vi "ui_loop_message_handling.vi"(8 "error in (no error)":errorcluster caption="错误输入（无错误）", 9 "UI Control Refs Cluster":T1 caption="UI控件引用簇", 10 "User Event - Stop":refnum<user-event>, 11 "UI Message Queue Ref":refnum<queue> caption="UI消息队列引用") -> (0 "error out":errorcluster caption="错误输出")   [LabVIEW 2015]
uses:
  support_vis/message_queue/message_cluster.ctl
  type_definitions/ui_data.ctl
  type_definitions/shared_variables.ctl
  globals/global_all_ui_loop_stop.vi
  globals/global_configuration_options.vi
  globals/global_ui_stream_and_variable_connections.vi
  support_vis/message_queue/message_queue.lvlib
  support_vis/user_event_stop/user_event_stop.lvlib
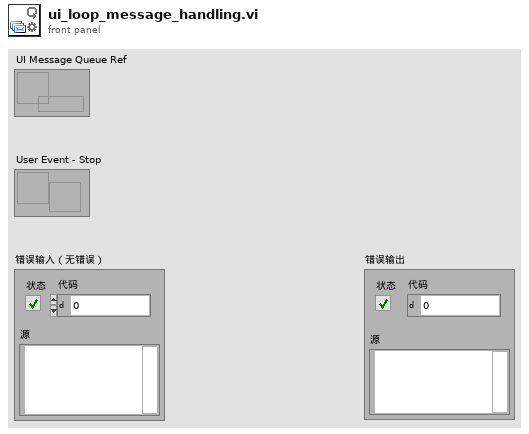
[diagram p1: front panel]
types:
  T1 = typedef "ui_data.ctl" = cluster{"Connected? Ref":refnum<vi>, "Controller Address Ref":refnum<vi>, "Error Infomation Ref":refnum<vi>, "Scan Engine Period (ms) Ref":refnum<vi>, "Number of Data Files Ref":refnum<vi>, "System Time Ref":refnum<vi>, "Free Memory Ref":refnum<vi>, "Device Tree Ref":refnum<vi>, "Controller Working Status Ref":refnum<vi>, "Connect to RT":refnum<vi>, "Exit":refnum<vi>, "Tab Ref":refnum<vi>, "Live Data Ref":refnum<vi>, "Resource Utilization (%) Ref":refnum<vi>}
  T2 = enum8{"Enabled", "Disabled", "Disabled and Grayed Out"}
  T3 = typedef "message_queue.lvlib/message_cluster.ctl" = cluster{"Message":string, "Message Data":variant}
  T4 = cluster{"Left Cell String":string, "Child Text":string[], "Child Tag":string, "Item Indent":i32, "Child Only?":bool, "Glyph Index":i32}[]
  T5 = typedef "shared_variables.ctl" = cluster{"System Time":timestamp, "CPU 1 Usage":dbl, "CPU 2 Usage":dbl, "Driver Space":dbl, "Free Memory":dbl, "Scan Engine Period (ms)":u32, "Number of Data Files":u32}
  T6 = cluster{"CPU 1 Usage":dbl, "CPU 2 Usage":dbl, "Driver Space":dbl}
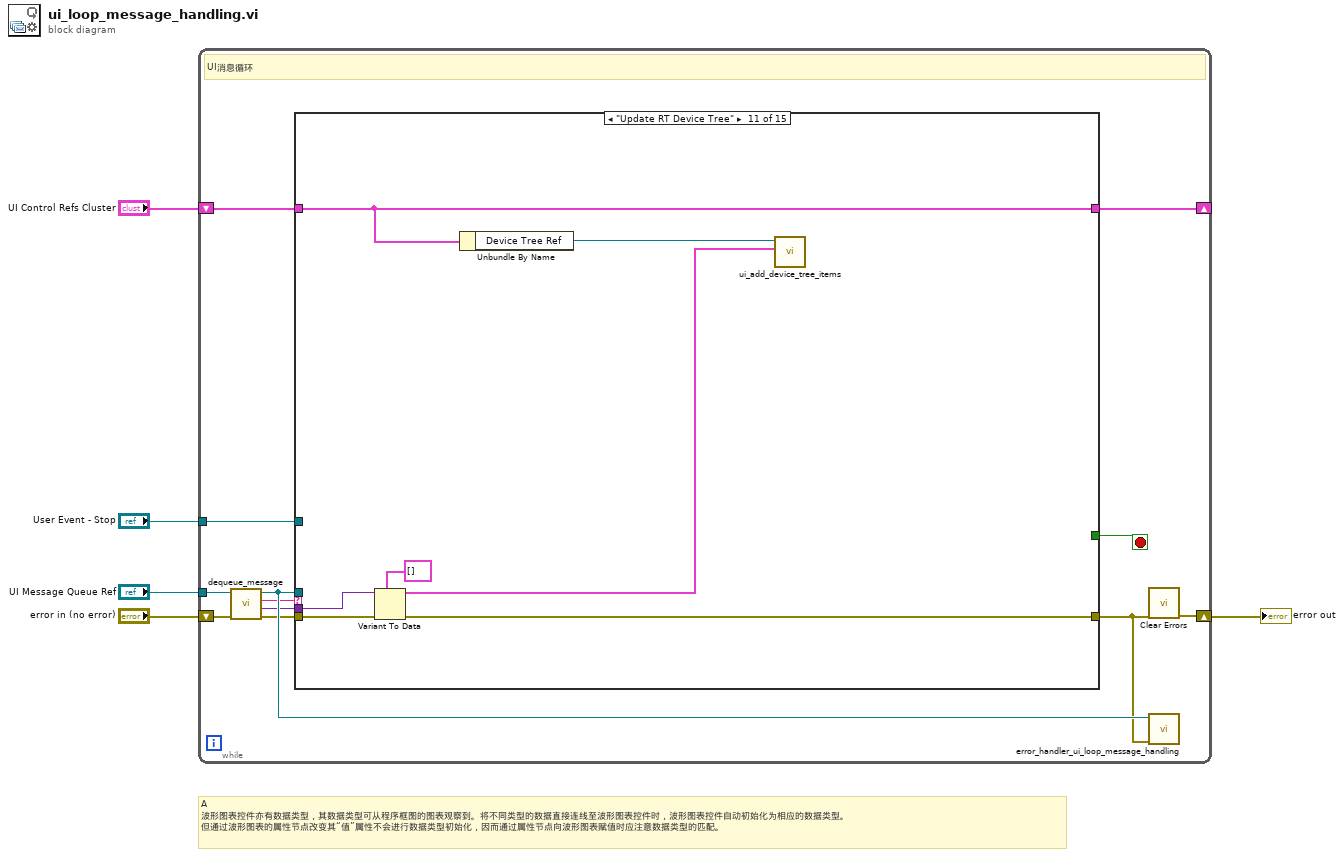
[diagram p0: block diagram]
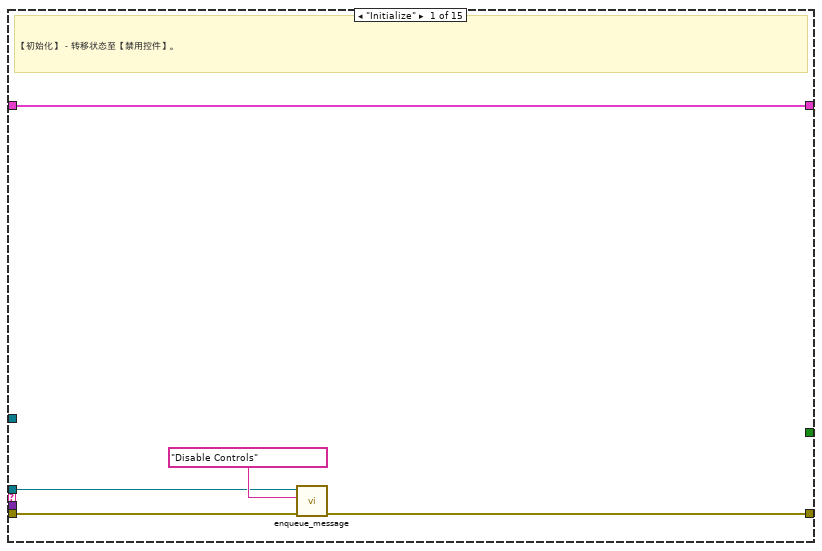
[diagram p2: hidden frame]
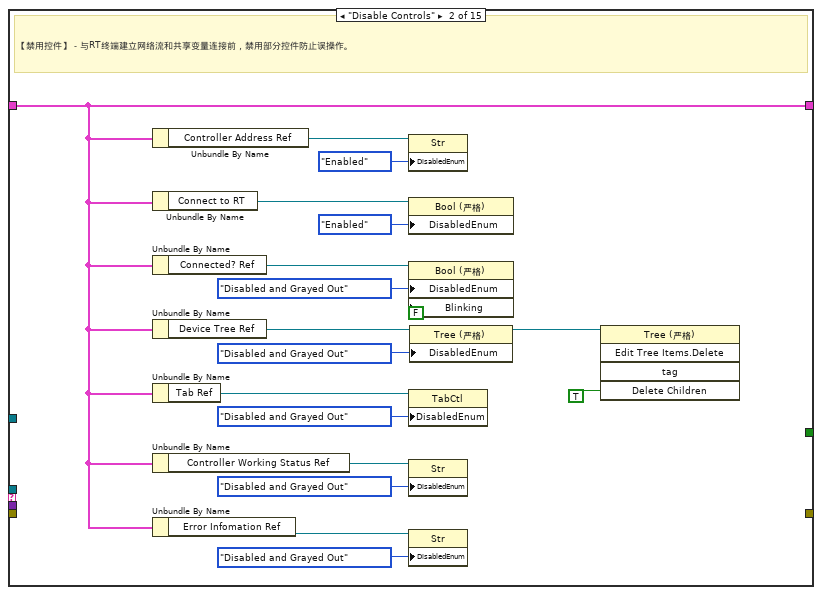
[diagram p3: hidden frame]
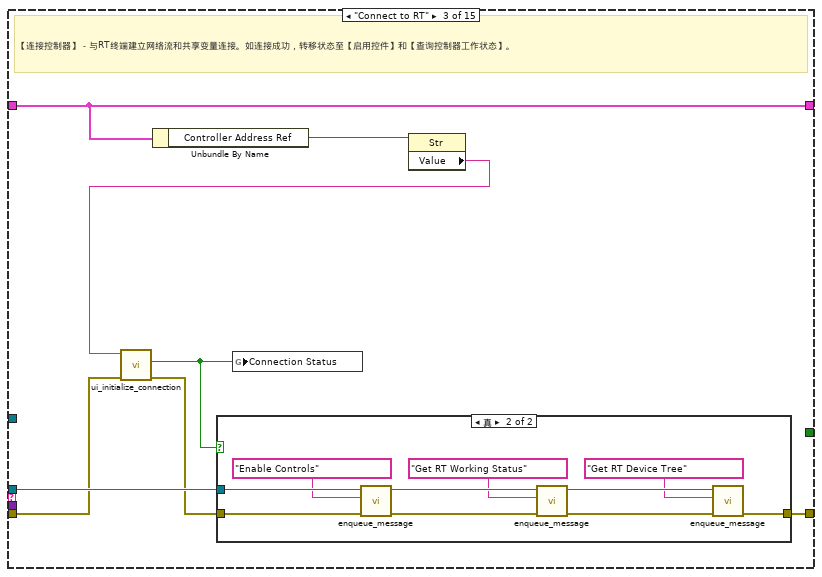
[diagram p4: hidden frame]
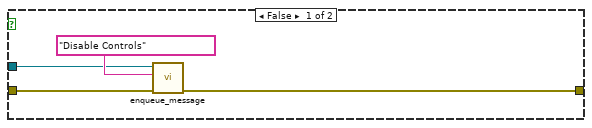
[diagram p5: hidden frame]
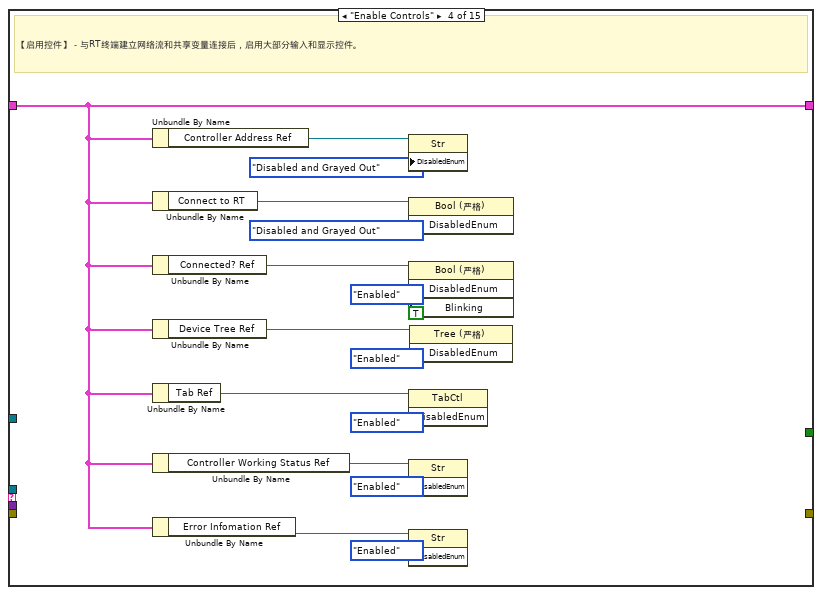
[diagram p6: hidden frame]
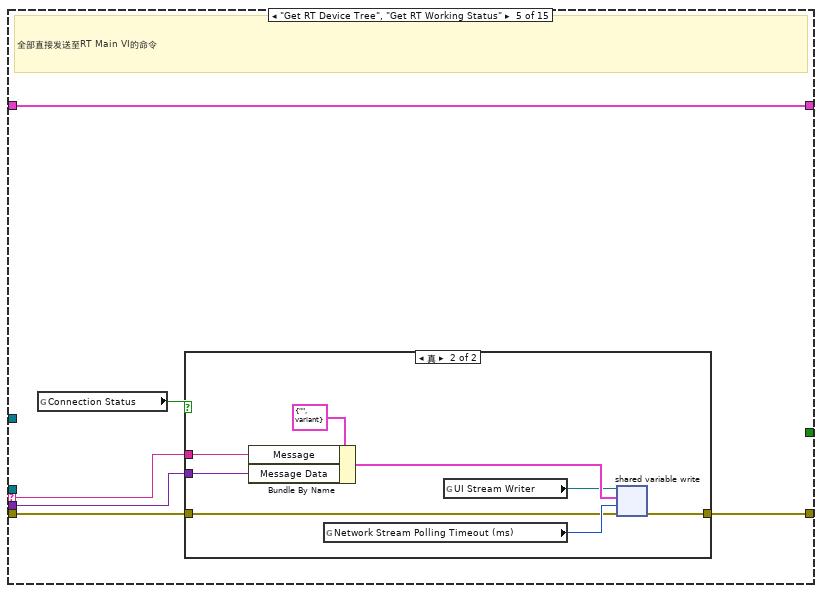
[diagram p7: hidden frame]
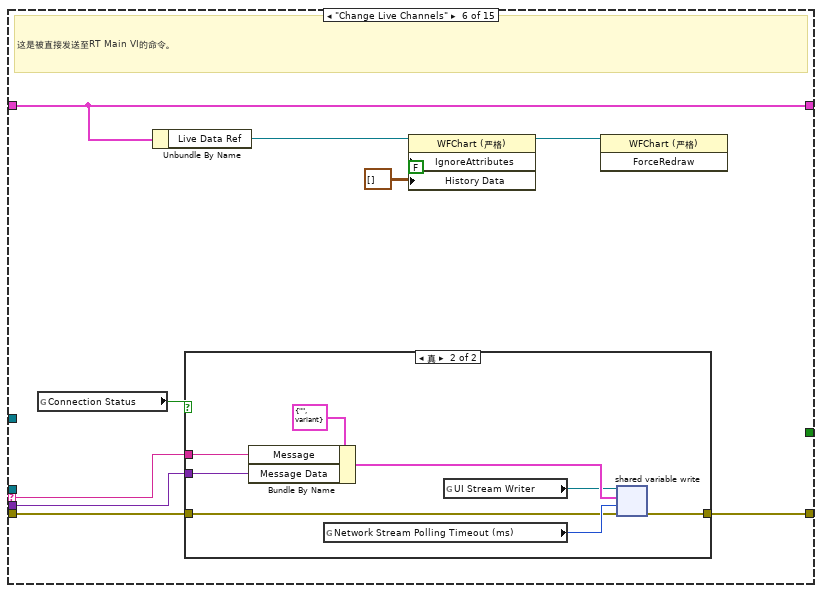
[diagram p9: hidden frame]
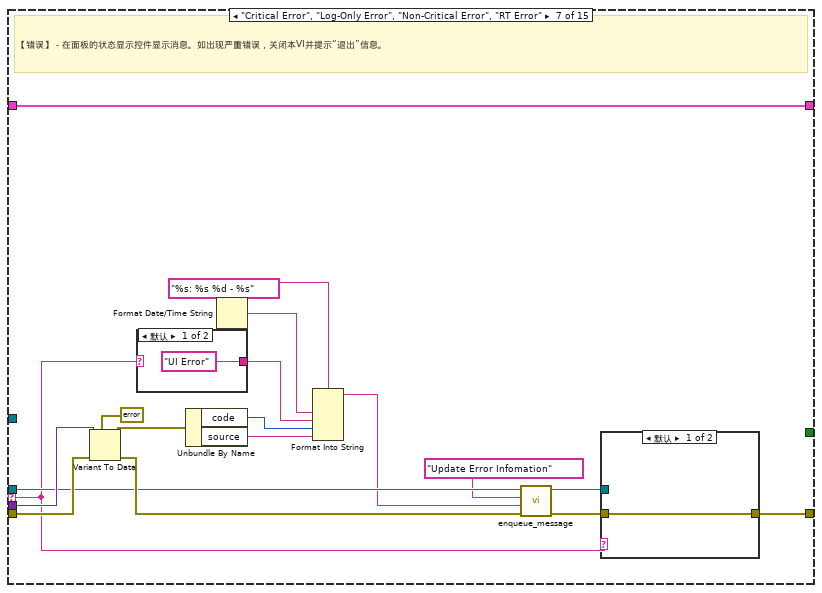
[diagram p11: hidden frame]
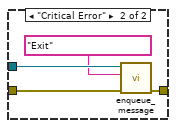
[diagram p13: hidden frame]
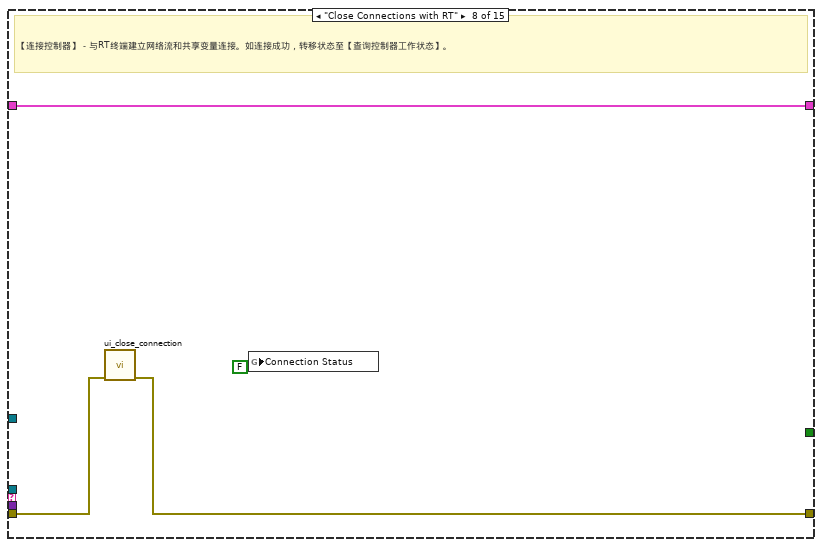
[diagram p14: hidden frame]
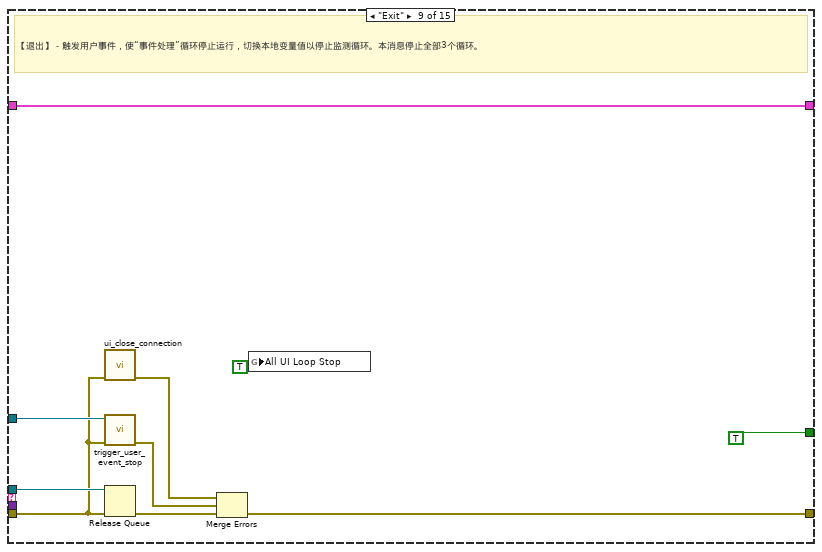
[diagram p15: hidden frame]
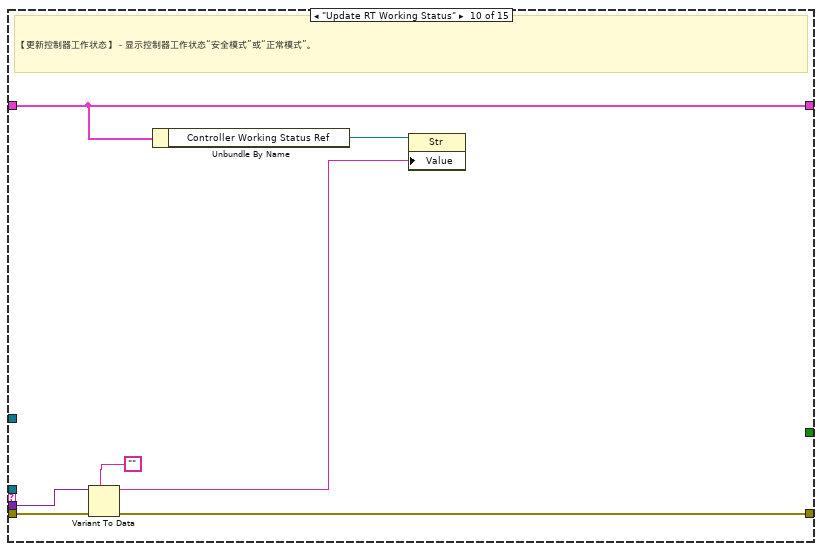
[diagram p16: hidden frame]
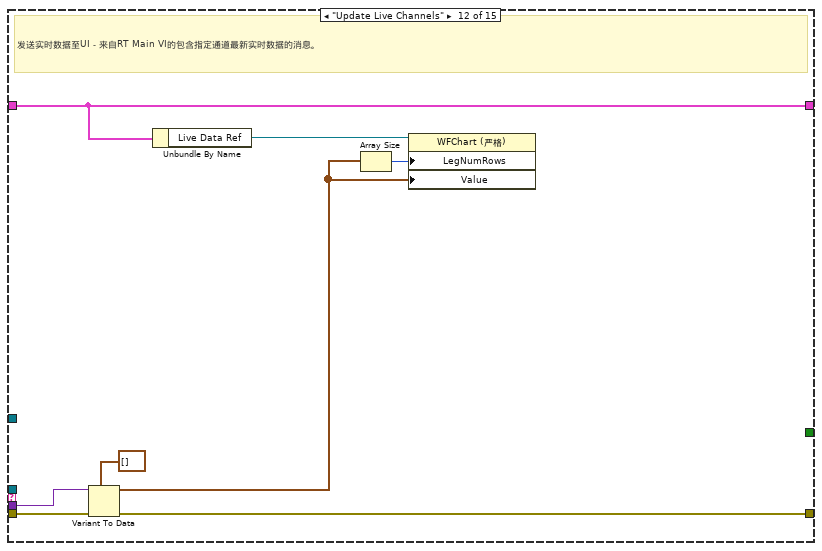
[diagram p17: hidden frame]
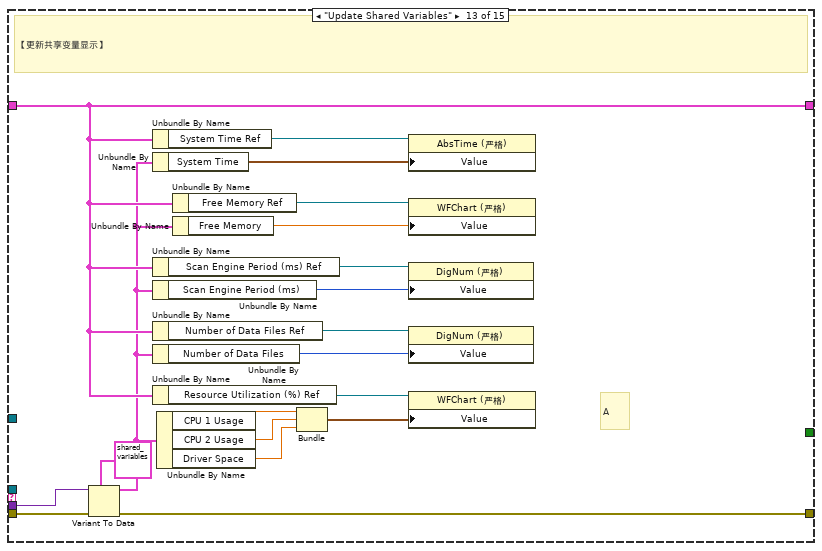
[diagram p18: hidden frame]
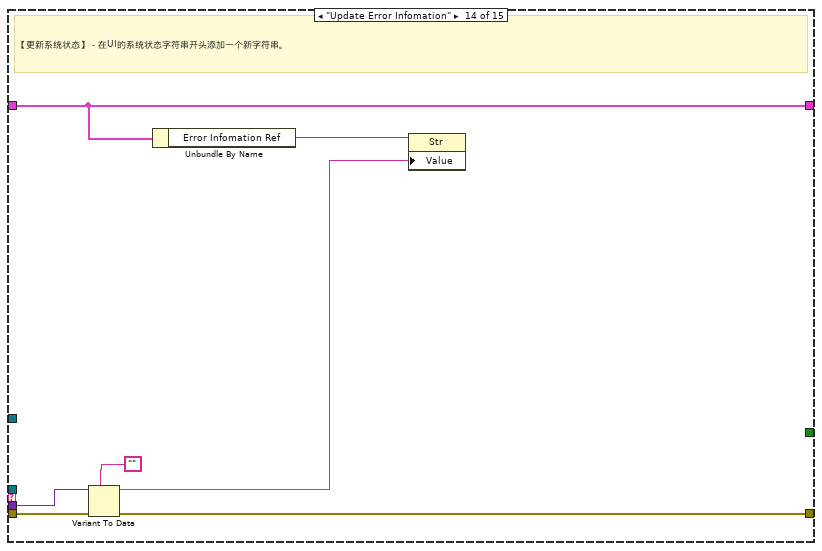
[diagram p19: hidden frame]
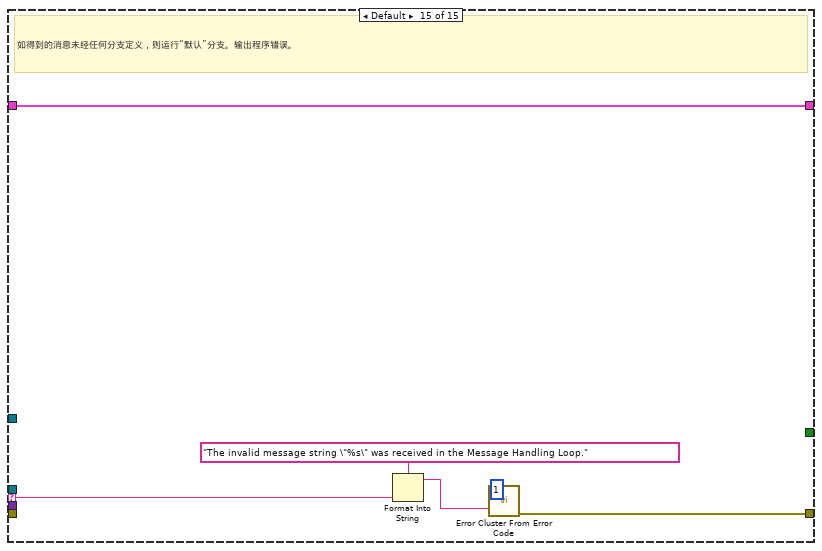
[diagram p20: hidden frame]
diagram:
  # "A\n波形图表控件亦有数据类型，其数据类型可从程序框图的图表观察到。将不同类型的数据直接连线至波形图表控件时，波形图表控件自动初始化为相应的数据类型。\n但通过波形图表的属性节点改变其“值”属性不会进行数据类型初始化，因而通过属性节点向波形图表赋值时应注意数据类型的匹配。"
  n1 = while {
    tunnel: "UI Message Queue Ref" -> [w10]
    tunnel: "User Event - Stop" -> [w15]
    shift-right: [w6] -> w1
    shift-left: "error in (no error)" -> [w14]
    shift-right: [w8] -> _
    shift-left: "UI Control Refs Cluster" -> [w9]
    stop <- w16 stop-if-true
    # "UI消息循环"
    n2 = call "dequeue_message.vi"("error in (no error)"=w14, "Message Queue"=w10) -> ("error out"=w13:errorcluster, "Message Data"=w11:variant, "Message"=w12:string, "dup Message Queue"=w17:refnum<queue>)  [unwired: 6 in]
    n3 = case "Message Cases" shown="\"Update RT Device Tree\"" w12 {
      selector: w12 -> [_ _ _ _ w81 w100 w114 _ _ _ _ _ _ _ w204]
      tunnel: w17 -> [w18 _ w45 _ _ _ w118 _ w146 _ _ _ _ _ _]
      tunnel: w13 -> [w21 _ w43 _ w84 w103 w128 w140 w144 w158 w164 w173 w192 w199 _]
      tunnel: [w19 _ w48 _ w83 w102 w129 w139 w150 w157 w163 w172 w191 w198 w202] -> w7
      tunnel: [_ _ _ _ _ _ _ _ TRUE _ _ _ _ _ _] -> w16
      tunnel: w11 -> [_ _ _ _ w82 w101 w126 _ _ w156 w162 w171 w190 w197 _]
      tunnel: w15 -> [_ _ _ _ _ _ _ _ w149 _ _ _ _ _ _]
      tunnel: w9 -> [w22 w25 w47 w63 w79 w98 w130 w141 w148 w154 w165 w169 w177 w195 w200]
      tunnel: [w22 w25 w47 w63 w79 w98 w130 w141 w148 w154 w165 w169 w177 w195 w200] -> w8
      frame "Initialize" {
        # "【初始化】－转移状态至【禁用控件】。"
        n4 = call "enqueue_message.vi"("error in (no error)"=w21, "Message"="Disable Controls", "Message Queue"=w18) -> ("error out"=w19:errorcluster)  [unwired: 7 in, 1 out]
      }
      frame "Disable Controls" {
        # "【禁用控件】－与RT终端建立网络流和共享变量连接前，禁用部分控件防止误操作。"
        n5 = Unbundle By Name(w25) -> ("Controller Address Ref"=w40:refnum<vi>)
        n6 = Unbundle By Name(w25) -> ("Connect to RT"=w37:refnum<vi>)
        n7 = Unbundle By Name(w25) -> ("Connected? Ref"=w36:refnum<vi>)
        n8 = Unbundle By Name(w25) -> ("Device Tree Ref"=w33:refnum<vi>)
        n9 = Unbundle By Name(w25) -> ("Tab Ref"=w30:refnum<vi>)
        n10 = Unbundle By Name(w25) -> ("Controller Working Status Ref"=w29:refnum<vi>)
        n11 = Unbundle By Name(w25) -> ("Error Infomation Ref"=w26:refnum<vi>)
        n12 = property class="Str"(reference=w40, "DisabledEnum"=T2."Enabled" ("禁用")) -> ()  [unwired: 1 in, 2 out]
        n13 = property class="Bool (严格)"(reference=w37, "DisabledEnum"=T2."Enabled" ("禁用")) -> ()  [unwired: 1 in, 2 out]
        n14 = property class="Bool (严格)"(reference=w36, "DisabledEnum"=T2."Disabled and Grayed Out" ("禁用"), "Blinking"=FALSE ("闪烁")) -> ()  [unwired: 1 in, 2 out]
        n15 = property class="TabCtl"(reference=w30, "DisabledEnum"=T2."Disabled and Grayed Out" ("禁用")) -> ()  [unwired: 1 in, 2 out]
        n16 = property class="Str"(reference=w29, "DisabledEnum"=T2."Disabled and Grayed Out" ("禁用")) -> ()  [unwired: 1 in, 2 out]
        n17 = property class="Str"(reference=w26, "DisabledEnum"=T2."Disabled and Grayed Out" ("禁用")) -> ()  [unwired: 1 in, 2 out]
        n18 = property class="Tree (严格)"(reference=w33, "DisabledEnum"=T2."Disabled and Grayed Out" ("禁用")) -> (reference out=w24:refnum<vi>)  [unwired: 1 in, 1 out]
        n19 = invoke class="Tree (严格)" method="Edit Tree Items.Delete"(reference=w24, "Delete Children"=TRUE ("删除子项？")) -> ()  [unwired: 3 in, 5 out]
      }
      frame "Connect to RT" {
        # "【连接控制器】－与RT终端建立网络流和共享变量连接。如连接成功，转移状态至【启用控件】和【查询控制器工作状态】。"
        n20 = Unbundle By Name(w47) -> ("Controller Address Ref"=w46:refnum<vi>)
        n21 = property class="Str"(reference=w46) -> ("Value"=w44:string)  [unwired: 1 in, 2 out]
        n22 = call "ui_initialize_connection.vi"("error in (no error)"=w43, "Controller Address"=w44) -> ("error out"=w42:errorcluster, "Connected?"=w41:bool)  [unwired: 8 in]
        n23 = case shown="真" w41 {
          tunnel: [w52 w56] -> w48
          tunnel: w45 -> [w50 w62]
          tunnel: w42 -> [w49 w61]
          frame False {
            n24 = call "enqueue_message.vi"("error in (no error)"=w49, "Message"="Disable Controls", "Message Queue"=w50) -> ("error out"=w52:errorcluster)  [unwired: 7 in, 1 out]
          }
          frame True {
            n25 = call "enqueue_message.vi"("error in (no error)"=w61, "Message"="Enable Controls", "Message Queue"=w62) -> ("error out"=w59:errorcluster, "dup Message Queue"=w60:refnum<queue>)  [unwired: 7 in]
            n26 = call "enqueue_message.vi"("error in (no error)"=w59, "Message"="Get RT Working Status", "Message Queue"=w60) -> ("error out"=w58:errorcluster, "dup Message Queue"=w57:refnum<queue>)  [unwired: 7 in]
            n27 = call "enqueue_message.vi"("error in (no error)"=w58, "Message"="Get RT Device Tree", "Message Queue"=w57) -> ("error out"=w56:errorcluster)  [unwired: 7 in, 1 out]
          }
        }
        n28 = global write "global_all_ui_loop_stop.vi" "Connection Status"(w41) -> ()
      }
      frame "Enable Controls" {
        # "【启用控件】－与RT终端建立网络流和共享变量连接后，启用大部分输入和显示控件。"
        n29 = Unbundle By Name(w63) -> ("Controller Address Ref"=w78:refnum<vi>)
        n30 = Unbundle By Name(w63) -> ("Connect to RT"=w75:refnum<vi>)
        n31 = Unbundle By Name(w63) -> ("Connected? Ref"=w74:refnum<vi>)
        n32 = Unbundle By Name(w63) -> ("Device Tree Ref"=w71:refnum<vi>)
        n33 = Unbundle By Name(w63) -> ("Tab Ref"=w68:refnum<vi>)
        n34 = Unbundle By Name(w63) -> ("Controller Working Status Ref"=w67:refnum<vi>)
        n35 = Unbundle By Name(w63) -> ("Error Infomation Ref"=w64:refnum<vi>)
        n36 = property class="Str"(reference=w78, "DisabledEnum"=T2."Disabled and Grayed Out" ("禁用")) -> ()  [unwired: 1 in, 2 out]
        n37 = property class="Bool (严格)"(reference=w75, "DisabledEnum"=T2."Disabled and Grayed Out" ("禁用")) -> ()  [unwired: 1 in, 2 out]
        n38 = property class="Bool (严格)"(reference=w74, "DisabledEnum"=T2."Enabled" ("禁用"), "Blinking"=TRUE ("闪烁")) -> ()  [unwired: 1 in, 2 out]
        n39 = property class="TabCtl"(reference=w68, "DisabledEnum"=T2."Enabled" ("禁用")) -> ()  [unwired: 1 in, 2 out]
        n40 = property class="Str"(reference=w67, "DisabledEnum"=T2."Enabled" ("禁用")) -> ()  [unwired: 1 in, 2 out]
        n41 = property class="Str"(reference=w64, "DisabledEnum"=T2."Enabled" ("禁用")) -> ()  [unwired: 1 in, 2 out]
        n42 = property class="Tree (严格)"(reference=w71, "DisabledEnum"=T2."Enabled" ("禁用")) -> ()  [unwired: 1 in, 2 out]
      }
      frame "Get RT Device Tree", "Get RT Working Status" {
        # "全部直接发送至RT Main VI的命令"
        n43 = global read "global_all_ui_loop_stop.vi" "Connection Status"() -> (w80:bool)
        n44 = case shown="真" w80 {
          tunnel: w84 -> [w85 w86]
          tunnel: [w85 w93] -> w83
          tunnel: w82 -> [_ w88]
          tunnel: w81 -> [_ w89]
          frame False {
          }
          frame True {
            n45 = Bundle By Name(cluster=T3 {"Message"="", "Message Data"=variant} ("Message Cluster"), "Message"=w89, "Message Data"=w88) -> (w90:T3)
            n46 = global read "global_configuration_options.vi" "Network Stream Polling Timeout (ms)"() -> (w92:i32)
            n47 = global read "global_ui_stream_and_variable_connections.vi" "UI Stream Writer"() -> (w87:refnum<k21>)
            n48 = shared-variable-write(w87, w86, w90, w92) -> (w93:errorcluster)  [unwired: 2 out]
          }
        }
      }
      frame "Change Live Channels" {
        # "这是被直接发送至RT Main VI的命令。"
        n49 = global read "global_all_ui_loop_stop.vi" "Connection Status"() -> (w99:bool)
        n50 = Unbundle By Name(w98) -> ("Live Data Ref"=w95:refnum<vi>)
        n51 = case shown="真" w99 {
          tunnel: w103 -> [w104 w105]
          tunnel: [w104 w112] -> w102
          tunnel: w101 -> [_ w107]
          tunnel: w100 -> [_ w108]
          frame False {
          }
          frame True {
            n52 = Bundle By Name(cluster=T3 {"Message"="", "Message Data"=variant} ("Message Cluster"), "Message"=w108, "Message Data"=w107) -> (w109:T3)
            n53 = global read "global_configuration_options.vi" "Network Stream Polling Timeout (ms)"() -> (w111:i32)
            n54 = global read "global_ui_stream_and_variable_connections.vi" "UI Stream Writer"() -> (w106:refnum<k21>)
            n55 = shared-variable-write(w106, w105, w109, w111) -> (w112:errorcluster)  [unwired: 2 out]
          }
        }
        n56 = property class="WFChart (严格)"(reference=w95, "IgnoreAttributes"=FALSE ("忽略属性"), "History Data"=waveform(dbl)[][] []) -> (reference out=w94:refnum<vi>)  [unwired: 1 in, 1 out]
        n57 = invoke class="WFChart (严格)" method="ForceRedraw"(reference=w94) -> ()  [unwired: 2 in, 3 out]
      }
      frame "Critical Error", "Log-Only Error", "Non-Critical Error", "RT Error" {
        # "【错误】－在面板的状态显示控件显示消息。如出现严重错误，关闭本VI并提示“退出”信息。"
        n58 = Variant To Data(error in=w128, type=errorcluster {"status"=FALSE, "code"=0, "source"=""} ("error constant"), Variant=w126) -> (data=w121:errorcluster, error out=w127:errorcluster)
        n59 = case shown="默认" w114 {
          selector: w114 -> [_ w132]
          tunnel: ["UI Error" w132] -> w113
          frame Default {
          }
          frame "RT Error" {
          }
        }
        n60 = Unbundle By Name(w121) -> ("code"=w120:i32, "source"=w124:string)
        n61 = Format Date/Time String() -> (date/time string=w123:string)  [unwired: 3 in]
        n62 = Format Into String(format string="%s: %s %d - %s", w123, w113, w120, w124) -> (resulting string=w115:string)  [unwired: 2 in, 1 out]
        n63 = call "enqueue_message.vi"("error in (no error)"=w127, "Message Data"=w115, "Message"="Update Error Infomation", "Message Queue"=w118) -> ("error out"=w119:errorcluster, "dup Message Queue"=w117:refnum<queue>)  [unwired: 6 in]
        n64 = case shown="默认" w114 {
          tunnel: w119 -> [w133 w137]
          tunnel: w117 -> [_ w135]
          tunnel: [w133 w136] -> w129
          frame Default {
          }
          frame "Critical Error" {
            n65 = call "enqueue_message.vi"("error in (no error)"=w137, "Message"="Exit", "Message Queue"=w135) -> ("error out"=w136:errorcluster)  [unwired: 7 in, 1 out]
          }
        }
      }
      frame "Close Connections with RT" {
        # "【连接控制器】－与RT终端建立网络流和共享变量连接。如连接成功，转移状态至【查询控制器工作状态】。"
        n66 = call "ui_close_connection.vi"("error in (no error)"=w140) -> ("error out"=w139:errorcluster)  [unwired: 10 in]
        n67 = global write "global_all_ui_loop_stop.vi" "Connection Status"(FALSE) -> ()
      }
      frame "Exit" {
        # "【退出】－触发用户事件，使“事件处理”循环停止运行，切换本地变量值以停止监测循环。本消息停止全部3个循环。"
        n68 = call "ui_close_connection.vi"("error in (no error)"=w144) -> ("error out"=w143:errorcluster)  [unwired: 10 in]
        n69 = call "trigger_user_event_stop.vi"("error in (no error)"=w144, "User Event - Stop"=w149) -> ("error out"=w142:errorcluster)  [unwired: 9 in]
        n70 = Release Queue(queue=w146, error in (no error)=w144) -> (error out=w147:errorcluster)  [unwired: 1 in, 2 out]
        n71 = Merge Errors(w143, w142, w147) -> (w150:errorcluster)
        n72 = global write "global_all_ui_loop_stop.vi" "All UI Loop Stop"(TRUE ("Stop Monitoring Loop")) -> ()
      }
      frame "Update RT Working Status" {
        # "【更新控制器工作状态】－显示控制器工作状态“安全模式”或“正常模式”。"
        n73 = Variant To Data(error in=w158, type="", Variant=w156) -> (data=w152:string, error out=w157:errorcluster)
        n74 = Unbundle By Name(w154) -> ("Controller Working Status Ref"=w153:refnum<vi>)
        n75 = property class="Str"(reference=w153, "Value"=w152) -> ()  [unwired: 1 in, 2 out]
      }
      frame "Update RT Device Tree" {
        n76 = Variant To Data(error in=w164, type=T4 [] ("Device Property Array"), Variant=w162) -> (data=w159:T4, error out=w163:errorcluster)
        n77 = Unbundle By Name(w165) -> ("Device Tree Ref"=w160:refnum<vi>)
        n78 = call "ui_add_device_tree_items.vi"("Device Tree Items"=w159, "Device Tree Ref"=w160) -> ()  [unwired: 10 in]
      }
      frame "Update Live Channels" {
        # "发送实时数据至UI－来自RT Main VI的包含指定通道最新实时数据的消息。"
        n79 = Variant To Data(error in=w173, type=waveform(dbl)[] [], Variant=w171) -> (data=w167:waveform(dbl)[], error out=w172:errorcluster)
        n80 = Unbundle By Name(w169) -> ("Live Data Ref"=w170:refnum<vi>)
        n81 = Array Size(array=w167) -> (size(s)=w166:i32)
        n82 = property class="WFChart (严格)"(reference=w170, "LegNumRows"=w166, "Value"=w167) -> ()  [unwired: 1 in, 2 out]
      }
      frame "Update Shared Variables" {
        # "A"
        # "【更新共享变量显示】"
        n83 = Variant To Data(error in=w192, type=T5 {"System Time"=timestamp(0 s since 1904-01-01), "CPU 1 Usage"=0.0, "CPU 2 Usage"=0.0, "Driver Space"=0.0, "Free Memory"=0.0, "Scan Engine Period (ms)"=0, "Number of Data Files"=0} ("Shared Variables"), Variant=w190) -> (data=w176:T5, error out=w191:errorcluster)
        n84 = Unbundle By Name(w177) -> ("System Time Ref"=w188:refnum<vi>)
        n85 = Unbundle By Name(w176) -> ("System Time"=w185:timestamp)
        n86 = Unbundle By Name(w177) -> ("Scan Engine Period (ms) Ref"=w181:refnum<vi>)
        n87 = Unbundle By Name(w176) -> ("Scan Engine Period (ms)"=w180:u32)
        n88 = Unbundle By Name(w177) -> ("Number of Data Files Ref"=w179:refnum<vi>)
        n89 = Unbundle By Name(w176) -> ("Number of Data Files"=w178:u32)
        n90 = Unbundle By Name(w177) -> ("Resource Utilization (%) Ref"=w184:refnum<vi>)
        n91 = Unbundle By Name(w176) -> ("CPU 1 Usage"=w187:dbl, "CPU 2 Usage"=w186:dbl, "Driver Space"=w174:dbl)
        n92 = Unbundle By Name(w177) -> ("Free Memory Ref"=w183:refnum<vi>)
        n93 = Unbundle By Name(w176) -> ("Free Memory"=w182:dbl)
        n94 = Bundle("CPU 1 Usage"=w187, "CPU 2 Usage"=w186, "Driver Space"=w174) -> (w175:T6)  [unwired: 1 in]
        n95 = property class="AbsTime (严格)"(reference=w188, "Value"=w185) -> ()  [unwired: 1 in, 2 out]
        n96 = property class="WFChart (严格)"(reference=w183, "Value"=w182) -> ()  [unwired: 1 in, 2 out]
        n97 = property class="DigNum (严格)"(reference=w181, "Value"=w180) -> ()  [unwired: 1 in, 2 out]
        n98 = property class="DigNum (严格)"(reference=w179, "Value"=w178) -> ()  [unwired: 1 in, 2 out]
        n99 = property class="WFChart (严格)"(reference=w184, "Value"=w175) -> ()  [unwired: 1 in, 2 out]
      }
      frame "Update Error Infomation" {
        # "【更新系统状态】－在UI的系统状态字符串开头添加一个新字符串。"
        n100 = Variant To Data(error in=w199, type="", Variant=w197) -> (data=w193:string, error out=w198:errorcluster)
        n101 = Unbundle By Name(w195) -> ("Error Infomation Ref"=w194:refnum<vi>)
        n102 = property class="Str"(reference=w194, "Value"=w193) -> ()  [unwired: 1 in, 2 out]
      }
      frame Default {
        # "如得到的消息未经任何分支定义，则运行“默认”分支。输出程序错误。"
        n103 = Format Into String(format string="The invalid message string \"%s\" was received in the Message Handling Loop." ("Invalid Message Loop Message"), w204) -> (resulting string=w201:string)  [unwired: 2 in, 1 out]
        n104 = call <vilib>:"Error Cluster From Error Code.vi"("error message (\"\")"=w201, "error code (0)"=1) -> ("error out"=w202:errorcluster)  [unwired: 7 in]
      }
    }
    n105 = call <vilib>:"Clear Errors.vi"("error in (no error)"=w7) -> ("error out"=w6:errorcluster)  [unwired: 5 in, 1 out]
    n106 = call "error_handler_ui_loop_message_handling.vi"("error in (no error)"=w7, "Message Queue"=w17) -> ()  [unwired: 9 in, 1 out]
  }
  "error out" <- w1
